vi "获取当前位置.vi"(8 "error in (no error)":errorcluster) -> (0 "error out":errorcluster, 2 "编码器计数值":u16, 3 "编码器工程量":dbl)   [LabVIEW 2016, in "elevator.lvlib"]
uses:
  elevator.lvlib
  DAM395CF/DAM395CF.lvlib
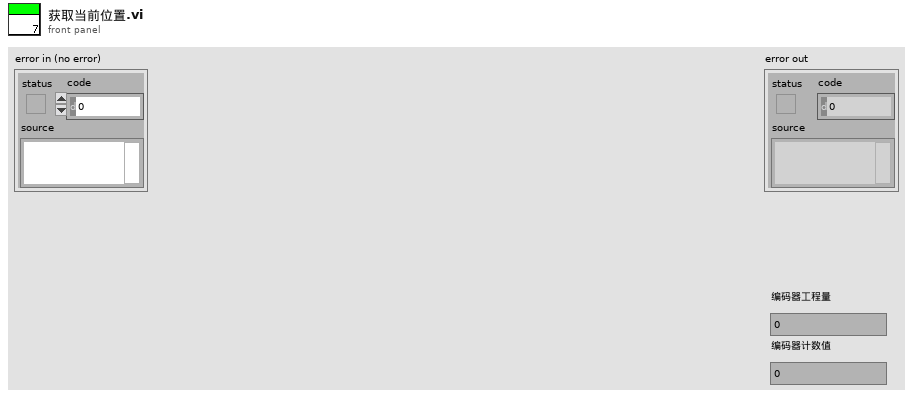
[diagram p1: front panel]
types:
  T1 = enum16{"通道0", "通道1", "通道2", "通道3", "通道4", "通道5", "通道6", "通道7"}
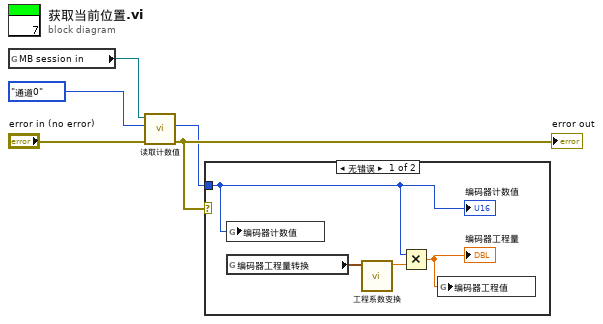
[diagram p0: block diagram]
diagram:
  n1 = global read "elevator 全局变量.vi" "MB session in"() -> (w5:refnum<class "MB_Master.lvclass">)
  n2 = call "读取计数值.vi"("error in (no error)"="error in (no error)", "通道"=T1."通道0", "MB session in"=w5) -> ("error out"=w2:errorcluster, "计数值"=w1:i32)  [unwired: 6 in, 1 out]
  "error out" <- w2
  n3 = case shown="无错误" w2 {
    tunnel: w1 -> [w7 _]
    frame No Error {
      n4 = global write "elevator 全局变量.vi" "编码器计数值"(w7) -> ()
      n5 = global read "elevator 全局变量.vi" "编码器工程量转换"() -> (w9:cluster{"编码器计数值":dbl, "工程计量值":dbl})
      n6 = call "工程系数变换.vi"("编码器工程量转换"=w9) -> ("工程变换系数"=w8:dbl)  [unwired: 10 in]
      n7 = Multiply(x=w7, y=w8) -> (x*y=w6:dbl)
      "编码器工程量" <- w6
      n8 = global write "elevator 全局变量.vi" "编码器工程值"(w6) -> ()
      "编码器计数值" <- w7
    }
    frame Error {
    }
  }
